vi "PH_DeformableMirror.Close.vi"(0 "VI in":refnum<vi>, 5 "error in (no error)":errorcluster) -> (14 "VI out":refnum<vi>, 19 "error out":errorcluster)   [LabVIEW 2014, in "PH_DeformableMirror.lvlib"]
uses:
  PH_DeformableMirror.lvlib
  CSlibraries-extern/shs/packages/dmdriver/DMirrorBase/DMirrorBase.lvclass
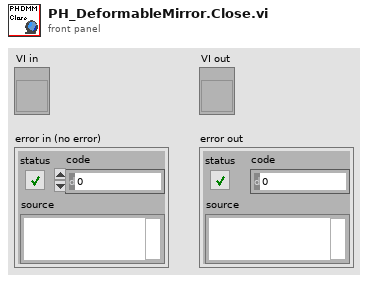
[diagram p1: front panel]
types:
  T1 = typedef "PH_DeformableMirror.lvlib/PH_DeformableMirror.i attribute.ctl" = cluster{"DMirror.lvlib:DMirrorBase.lvclass":refnum<class "DMirrorBase.lvclass">, "Device error":errorcluster, "GUI Refs":cluster{"Delete":refnum<vi>, "Device Error":refnum<vi>, "HV on":refnum<vi>, "Channel":refnum<vi>, "Voltage":refnum<vi>, "Channel Voltages":refnum<vi>}}
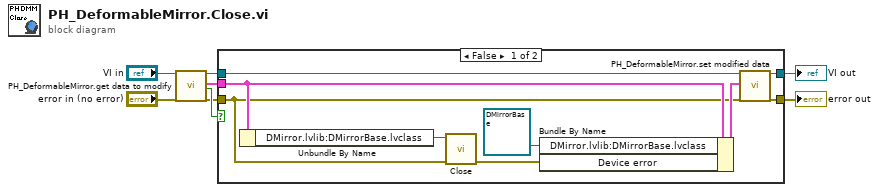
[diagram p0: block diagram]
diagram:
  n1 = call "PH_DeformableMirror.get data to modify.vi"("i ref in"="VI in", "error in (no error)"="error in (no error)") -> ("i ref out"=w3:refnum<vi>, "i attribute"=w8:T1, "timed out"=w7:bool, "error out"=w5:errorcluster)  [unwired: 14 in]
  n2 = case shown="False" w7 {
    tunnel: w3 -> [w17 w19]
    tunnel: [w16 w19] -> w4
    tunnel: w5 -> [w12 w18]
    tunnel: [w15 w18] -> w6
    tunnel: w8 -> [w13 _]
    frame False {
      n3 = Unbundle By Name(w13) -> ("DMirror.lvlib:DMirrorBase.lvclass"=w11:refnum<class "DMirrorBase.lvclass">)
      n4 = call-dynamic "Close.vi"("error in (no error)"=w12, "DMirrorBase in"=w11) -> ("error out"=w10:errorcluster)  [unwired: 9 in]
      n5 = Bundle By Name(cluster=w13, "DMirror.lvlib:DMirrorBase.lvclass"=refnum<class "DMirrorBase.lvclass"> refnum, "Device error"=w10) -> (w14:T1)
      n6 = call "PH_DeformableMirror.set modified data.vi"("i ref in"=w17, "i attribute"=w14, "error in (no error)"=w12) -> ("i ref out"=w16:refnum<vi>, "error out"=w15:errorcluster)  [unwired: 15 in]
    }
    frame True {
    }
  }
  "error out" <- w6
  "VI out" <- w4
